vi "Register for Result Events.vi"(8 "error in (no error)":errorcluster, 11 "Result Collector In":refnum<class "Result Collector.lvclass">) -> (0 "error out":errorcluster, 2 "Result Events":refnum<event-registration>, 3 "Result Collector Out":refnum<class "Result Collector.lvclass">)   [LabVIEW 2020, in "Result Collector.lvclass"]
uses:
  Result Collector.lvclass
  Result Types/Method Result/Method Result.ctl
  Result Types/Assertion Result/Public/TypeDefs/Status.ctl
  Result Types/Assertion Result/Assertion Result.ctl
  Result Types/Assertion Result/Public/TypeDefs/Assertion Type.ctl
  Result Types/Case Result/Test Case Result.ctl
  Result Types/Suite Results/Test Suite Result.ctl
  Result Collector.lvclass/Result Collector.ctl
  Result Types/Assertion Result/Assertion Result.lvlib
  Result Types/Method Result/Method Result.lvlib
  Result Types/Case Result/Test Case Result.lvlib
  Result Types/Suite Results/Test Suite Result.lvlib
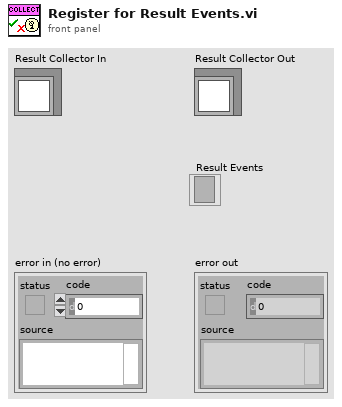
[diagram p1: front panel]
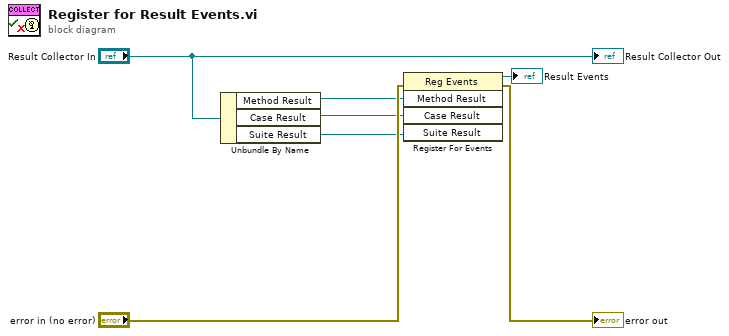
[diagram p0: block diagram]
diagram:
  n1 = Unbundle By Name("Result Collector In") -> ("Method Result"=w4:refnum<user-event>, "Case Result"=w3:refnum<user-event>, "Suite Result"=w2:refnum<user-event>)
  n2 = register-events(error in="error in (no error)", w4, w3, w2) -> (reference out=→"Result Events":refnum<event-registration>, error out=→"error out":errorcluster)  [unwired: 1 in]
  "Result Collector Out" <- "Result Collector In"
